vi "探头测量值显示.vi"(11 "校准参数":u16(ring) caption="校准参数：" items=["pH", "DO", "浊度", "电导率", "叶绿素a", "藻密度", "ORP", "COD", "DO2", "氯化物", "氨氮"]) -> (0 "线性系数":cluster{bool, "K":sgl, "B":sgl}, 1 "信号值":sgl, 2 "检测值":sgl, 3 "序列号":string, 4 "检测值.格式字符串":string, 5 "温度补偿系数":cluster{bool, "温度补偿系数":sgl}, 6 "信号值.格式字符串":string, 7 "电极状态标志":u16)   [LabVIEW 2016, in "斯坦道多参数.lvlib"]
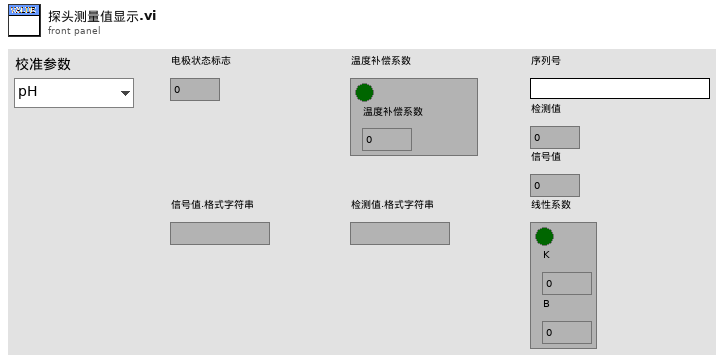
[diagram p1: front panel]
types:
  T1 = typedef "斯坦道多参数.lvlib/探头类型.ctl" = enum16{"禹山", "国弘", "纳清", "STD"}
  T2 = cluster{"pH探头选择":T1, "DO探头选择":T1, "电导率探头选择":T1, "浊度探头选择":T1, "叶绿素a探头选择":T1, "蓝绿藻探头选择":T1, "orp探头选择":T1, "COD探头选择":T1, "DO2探头选择":T1, "氨氮探头选择":T1, "水中油探头选择":T1}
  T3 = enum16{"null", "pH", "DO", "浊度", "电导率", "叶绿素a", "DO2"}
  T4 = enum16{"null", "pH", "DO", "浊度", "电导率", "叶绿素a", "DO2", "藻密度"}
  T5 = cluster{"输出值":cluster{"K":sgl, "B":sgl}, "SN":string}
  T6 = cluster{"电极状态标志":u16, "电极型号标志":u16, "酸碱度测量值":sgl, "温度测量值":sgl, "酸碱度信号值":sgl, "温度信号值":sgl, "酸碱度偏移修正值":sgl, "温度偏移修正值":sgl, "手动温度补偿值":sgl, "酸碱度电极零点":sgl, "酸碱度电极斜率":sgl, "第1点标准值记录":sgl, "第1点信号值记录":sgl, "第1点温度值记录":sgl, "第2点标准值记录":sgl, "第2点信号值记录":sgl, "第2点温度值记录":sgl, "命令滤波设定":u16, "温度模式":enum16{"ATC", "MTC"}, "生产批次":u16, "电极序号":u16, "串口地址":u16, "串口波特率":enum16{"9600", "19200", "115200"}, "串口校验位":enum16{"NONE", "ODD", "EVEN"}, "串口停止位":enum16{"1bit", "2bit"}, "第一点标准值":sgl, "第二点标准值":sgl}
  T7 = cluster{"报警码":u16, "pH数值":sgl, "0X0003_NC":sgl, "温度数据":sgl, "pH原始信号 mv":sgl, "0X0009_NC":string, "产品名称":string, "序列号":string, "硬件版本":string, "软件版本":string, "通讯地址":u16, "波特率":u16, "设备类型":u16, "0X0026_NC":string, "第一点原始数据":sgl, "第一点校准数据":sgl, "第二点原始数据":sgl, "第二点校准数据":sgl, "探头校准命令":u16, "温度校准参数":sgl, "温度校准命令":u16}
  T8 = cluster{"电极状态标志":u16, "电极型号标志":u16, "溶解氧测量值":sgl, "温度测量值":sgl, "溶解氧饱和度值":sgl, "盐度补偿值":sgl, "大气压补偿值":sgl, "溶解氧偏移修正值":sgl, "温度偏移修正值":sgl, "手动温度补偿值":sgl, "溶解氧电极零点":sgl, "溶解氧电极斜率":sgl, "第1点标准值记录":sgl, "第1点信号值记录":sgl, "第1点温度值记录":sgl, "第2点标准值记录":sgl, "第2点信号值记录":sgl, "第2点温度值记录":sgl, "命令滤波设定":u16, "温度模式":enum16{"ATC", "MTC"}, "生产批次":u16, "电极序号":u16, "串口地址":u16, "串口波特率":enum16{"9600", "19200", "115200"}, "串口校验位":enum16{"NONE", "ODD", "EVEN"}, "串口停止位":enum16{"1bit", "2bit"}, "第一点标准值":sgl, "第二点标准值":sgl}
  T9 = cluster{"报警码":u16, "溶解氧数值（mg/L）":sgl, "溶解氧数据（%）":sgl, "温度数据":sgl, "溶解氧原始信号 nA":sgl, "大气压力":sgl, "盐度":sgl, "0X0009_NC":string, "产品名称":string, "序列号":string, "硬件版本":string, "软件版本":string, "通讯地址":u16, "波特率":u16, "设备类型":u16, "0X0026_NC":string, "第一点原始数据":sgl, "第一点校准数据":sgl, "第二点原始数据":sgl, "第二点校准数据":sgl, "探头校准命令":u16, "温度校准参数":sgl, "温度校准命令":u16}
  T10 = cluster{"电极状态标志":u16, "电极型号标志":u16, "浊度测量值":sgl, "温度测量值":sgl, "浊度信号值":sgl, "浊度偏移修正值":sgl, "温度偏移修正值":sgl, "手动温度补偿值":sgl, "浊度电极零点":sgl, "浊度电极斜率":sgl, "清洁周期":u16, "命令滤波设定":u16, "温度模式":enum16{"ATC", "MTC"}, "生产批次":u16, "电极序号":u16, "串口地址":u16, "串口波特率":enum16{"9600", "19200", "115200"}, "串口校验位":enum16{"NONE", "ODD", "EVEN"}, "串口停止位":enum16{"1bit", "2bit"}, "第一点标准值":sgl, "第二点标准值":sgl, "第三点标准值":sgl}
  T11 = cluster{"报警码":u16, "浊度数值 NTU":sgl, "温度数据":sgl, "原始光强数值":u16, "量程":u16, "平均次数":u16, "清扫模式":u16, "清扫次数":u16, "清扫间隔分钟":u16, "0X000B_NC":string, "产品名称":string, "序列号":string, "硬件版本":string, "软件版本":string, "通讯地址":u16, "波特率":u16, "设备类型":u16, "0X0026_NC":string, "校准量程":u16, "第一点原始光强":u16, "第一点校准数据":sgl, "第二点原始光强":u16, "第二点校准数据":sgl, "第三点原始光强":u16, "第三点校准数据":sgl, "探头校准命令":u16, "温度校准参数":sgl, "温度校准命令":u16}
  T12 = cluster{"电极状态标志":u16, "电极型号标志":u16, "电导率测量值":sgl, "温度测量值":sgl, "电导率信号值":sgl, "温度信号值":sgl, "温度补偿系数":sgl, "电导率偏移修正值":sgl, "温度偏移修正值":sgl, "手动温度补偿值":sgl, "电导率电极零点":sgl, "电导率电极斜率":sgl, "命令滤波设定":u16, "温度模式":enum16{"ATC", "MTC"}, "生产批次":u16, "电极序号":u16, "串口地址":u16, "串口波特率":enum16{"9600", "19200", "115200"}, "串口校验位":enum16{"NONE", "ODD", "EVEN"}, "串口停止位":enum16{"1bit", "2bit"}, "第一点标准值":sgl, "第二点标准值":sgl}
  T13 = cluster{"报警码":u16, "电导率数据（uS/cm）":sgl, "0x0003 NC":sgl, "温度数据":sgl, "电导率原始信号电阻":sgl, "当前量程":u16, "温度补偿系数":sgl, "0X0009_NC":string, "产品名称":string, "序列号":string, "硬件版本":string, "软件版本":string, "通讯地址":u16, "波特率":u16, "设备类型":u16, "0X0026_NC":string, "第一点原始数据":sgl, "第一点校准数据":sgl, "0X0035_NC":sgl, "0X0037_NC":sgl, "探头校准命令":u16, "温度校准参数":sgl, "温度校准命令":u16}
  T14 = cluster{"报警码":u16, "叶绿素a":sgl, "温度数据":sgl, "原始光强数值":u16, "量程":u16, "平均次数":u16, "清扫模式":u16, "清扫次数":u16, "清扫间隔分钟":u16, "0X000B_NC":string, "产品名称":string, "序列号":string, "硬件版本":string, "软件版本":string, "通讯地址":u16, "波特率":u16, "设备类型":u16, "0X0026_NC":string, "校准量程":u16, "第一点原始光强":u16, "第一点校准数据":sgl, "第二点原始光强":u16, "第二点校准数据":sgl, "第三点原始光强":u16, "第三点校准数据":sgl, "探头校准命令":u16, "温度校准参数":sgl, "温度校准命令":u16}
  T15 = cluster{"报警码":u16, "蓝绿藻":sgl, "温度数据":sgl, "原始光强数值":u16, "量程":u16, "平均次数":u16, "清扫模式":u16, "清扫次数":u16, "清扫间隔分钟":u16, "0X000B_NC":string, "产品名称":string, "序列号":string, "硬件版本":string, "软件版本":string, "通讯地址":u16, "波特率":u16, "设备类型":u16, "0X0026_NC":string, "校准量程":u16, "第一点原始光强":u16, "第一点校准数据":sgl, "第二点原始光强":u16, "第二点校准数据":sgl, "第三点原始光强":u16, "第三点校准数据":sgl, "探头校准命令":u16, "温度校准参数":sgl, "温度校准命令":u16}
  T16 = cluster{"电极状态标志":u16, "电极型号标志":u16, "测量值":sgl, "温度测量值":sgl, "信号值":sgl, "温度信号值":sgl, "000AH_NC":sgl, "偏移修正值":sgl, "温度偏移修正值":sgl, "手动温度补偿值":sgl, "命令滤波设定":u16, "温度模式":enum16{"ATC", "MTC"}, "生产批次":u16, "传感器序号":u16, "串口地址":u16, "串口波特率":enum16{"9600", "19200", "115200"}, "串口校验位":enum16{"NONE", "ODD", "EVEN"}, "串口停止位":enum16{"1bit", "2bit"}}
  T17 = cluster{"电极状态标志":u16, "电极型号标志":u16, "COD测量值":sgl, "浊度测量值":sgl, "COD信号值":sgl, "浊度信号值":sgl, "温度测量值":sgl, "COD偏移修正值":sgl, "浊度偏移修正值":sgl, "COD水样校正值":sgl, "温度偏移修正值":sgl, "COD零点系数":sgl, "COD斜率系数":sgl, "浊度零点系数":sgl, "浊度斜率系数":sgl, "COD测值K值":sgl, "浊度测值K值":sgl, "浊度补偿COD系数值":sgl, "COD温度补偿系数值 ":sgl, "测量周期":u16, "清洗周期":u16, "命令寄存器":u16, "数字滤波设定":u16, "温度模式":enum16{"AUTO", "OFF"}, "生产批次":u16, "电极序号":u16, "串口地址":u16, "串口波特率":enum16{"9600", "19200", "115200"}, "串口校验位":enum16{"NONE", "ODD", "EVEN"}, "串口停止位":enum16{"1bit", "2bit"}, "第一点校正指令":u16, "第一点标准值":sgl, "第二点校正指令":u16, "第二点标准值":sgl, "第三点校正指令":u16, "第三点标准值":sgl, "COD吸光度":sgl, "浊度吸光度":sgl, "温度信号值":sgl}
  T18 = cluster{"电极状态标志":u16, "电极型号标志":u16, "测量值":sgl, "温度测量值":sgl, "信号值":sgl, "温度信号值":sgl, "偏移修正值":sgl, "温度偏移修正值":sgl, "手动温度补偿值":sgl, "电极零点":sgl, "电极斜率":sgl, "第1点标准值记录":sgl, "第1点信号值记录":sgl, "第1点温度值记录":sgl, "第2点标准值记录":sgl, "第2点信号值记录":sgl, "第2点温度值记录":sgl, "命令滤波设定":u16, "温度模式":enum16{"ATC", "MTC"}, "生产批次":u16, "电极序号":u16, "串口地址":u16, "串口波特率":enum16{"9600", "19200", "115200"}, "串口校验位":enum16{"NONE", "ODD", "EVEN"}, "串口停止位":enum16{"1bit", "2bit"}, "第一点标准值":sgl, "第二点标准值":sgl}
  T19 = cluster{"报警码":u16, "参数1数据":sgl, "参数2数据":sgl, "参数3数据":sgl, "参数4数据":sgl, "温度数据":sgl, "参数1原始信号":sgl, "参数2原始信号":sgl, "参数3原始信号":sgl, "参数4原始信号":sgl, "序列号":string, "硬件版本":string, "软件版本":string, "通讯地址":u16, "波特率":u16, "设备类型":u16, "0X0026_NC":string, "校准参数类型":u16, "第一点原始数据":sgl, "第一点校准数据":sgl, "第二点原始数据":sgl, "第二点校准数据":sgl, "探头校准命令":u16, "温度校准参数":sgl, "温度校准命令":u16}
  T20 = cluster{"电极状态标志":u16, "电极型号标志":u16, "测量值":sgl, "温度测量值":sgl, "信号值":sgl, "水中油B值":sgl, "温度B值":sgl, "水中油零点系数":sgl, "水中油斜率系数":sgl, "水中油K值":sgl, "空白电位值":sgl, "温度信号值":sgl, "温度补偿系数":sgl, "测量档位":u16, "清洁周期":u16, "命令寄存器":u16, "数位滤波设定":u16, "温度模式":enum16{"ATC", "MTC"}, "生产批次":u16, "电极序号":u16, "串口地址":u16, "串口波特率":enum16{"9600", "19200", "115200"}, "串口校验位":enum16{"NONE", "ODD", "EVEN"}, "串口停止位":enum16{"1bit", "2bit"}, "第一点校正指令":u16, "第一点标准值":sgl, "第二点校正指令":u16, "第二点标准值":sgl, "第三点校正指令":u16, "第三点标准值":sgl}
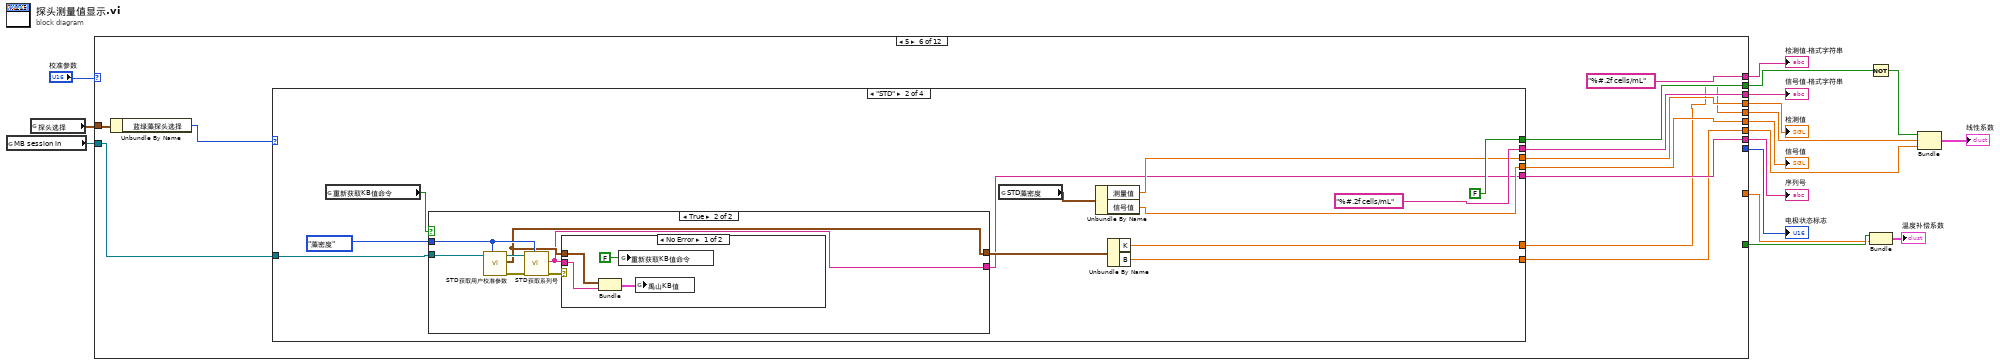
[diagram p0: block diagram]
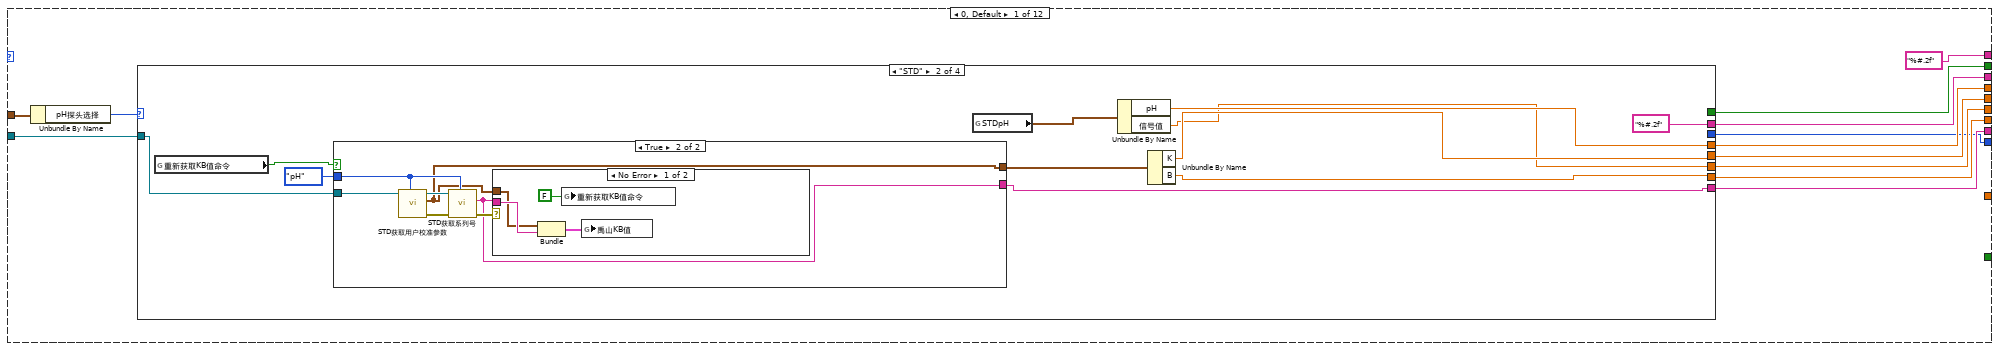
[diagram p2: hidden frame]
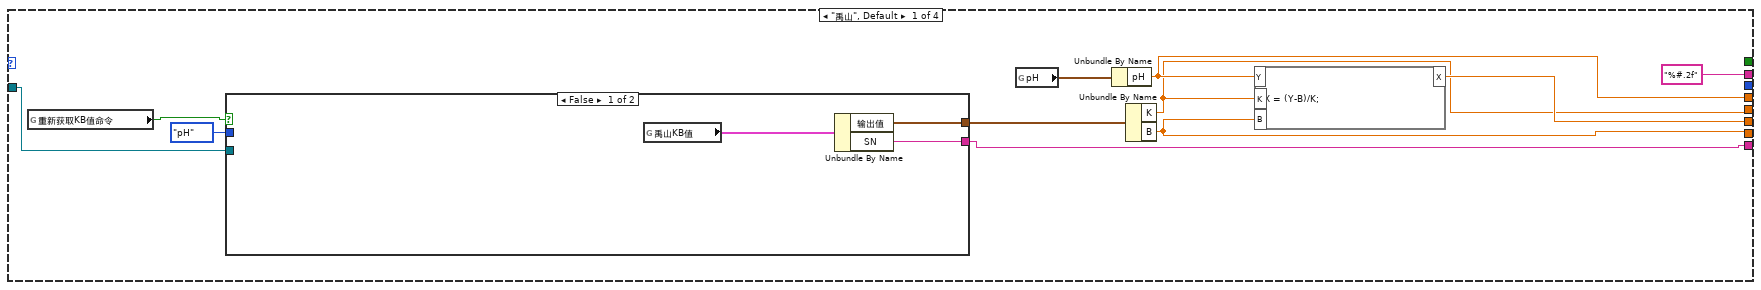
[diagram p3: hidden frame]
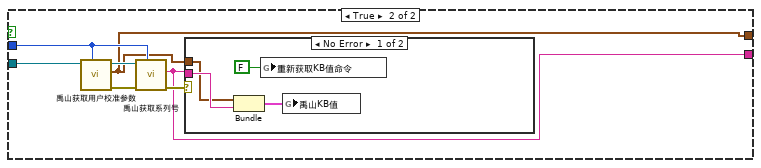
[diagram p4: hidden frame]
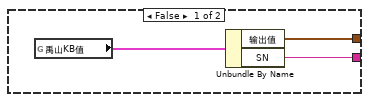
[diagram p6: hidden frame]
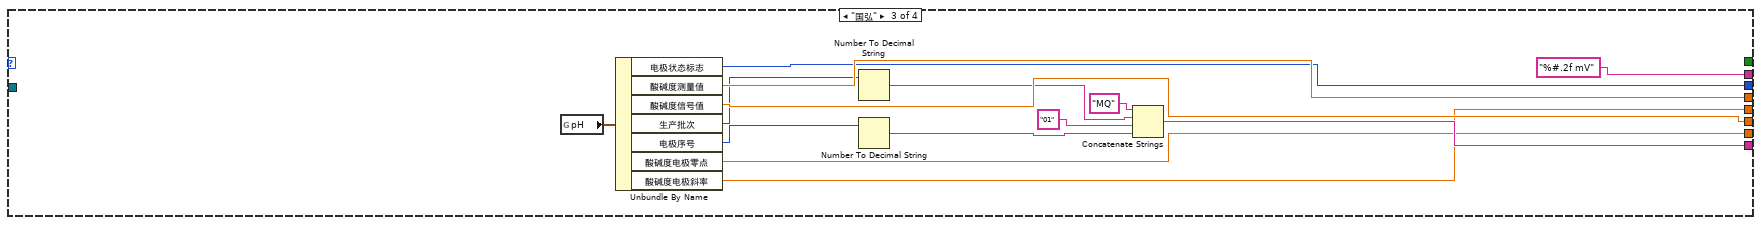
[diagram p8: hidden frame]
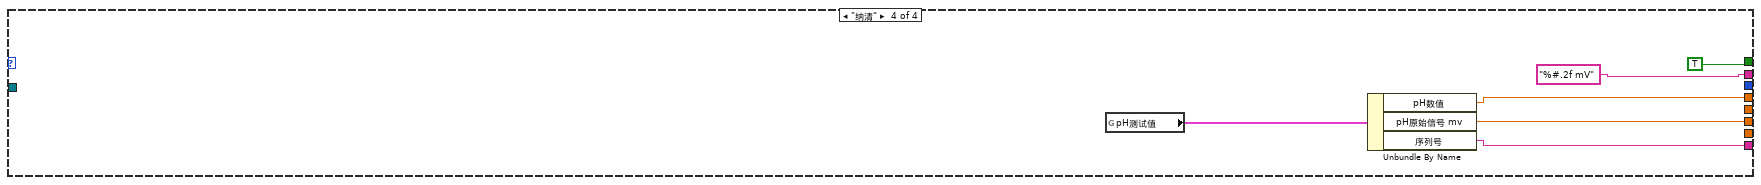
[diagram p9: hidden frame]
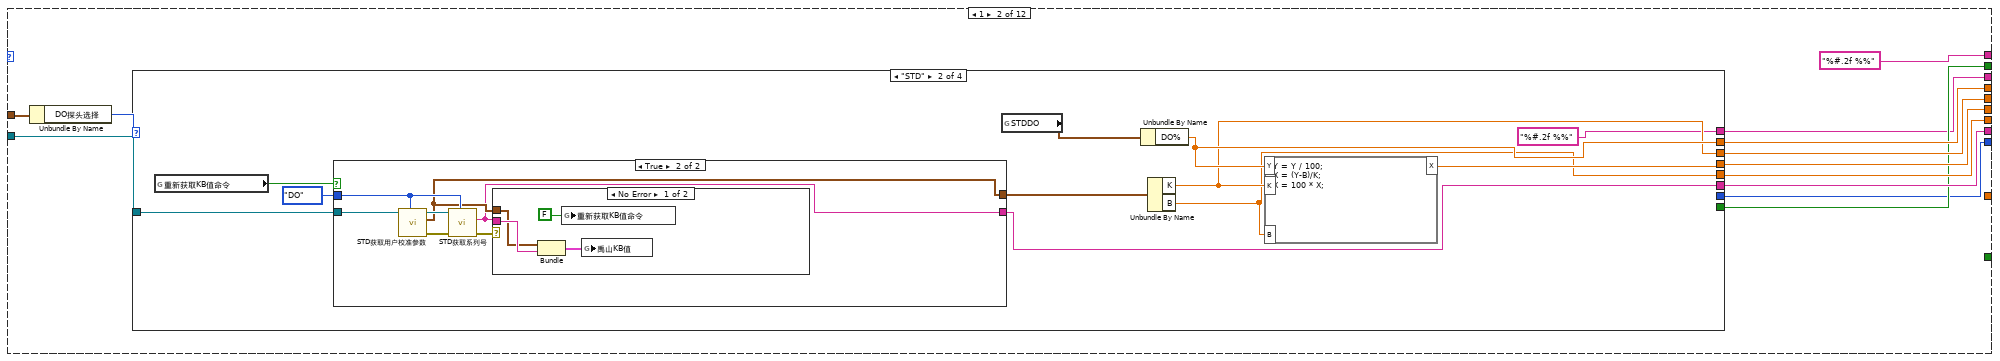
[diagram p10: hidden frame]
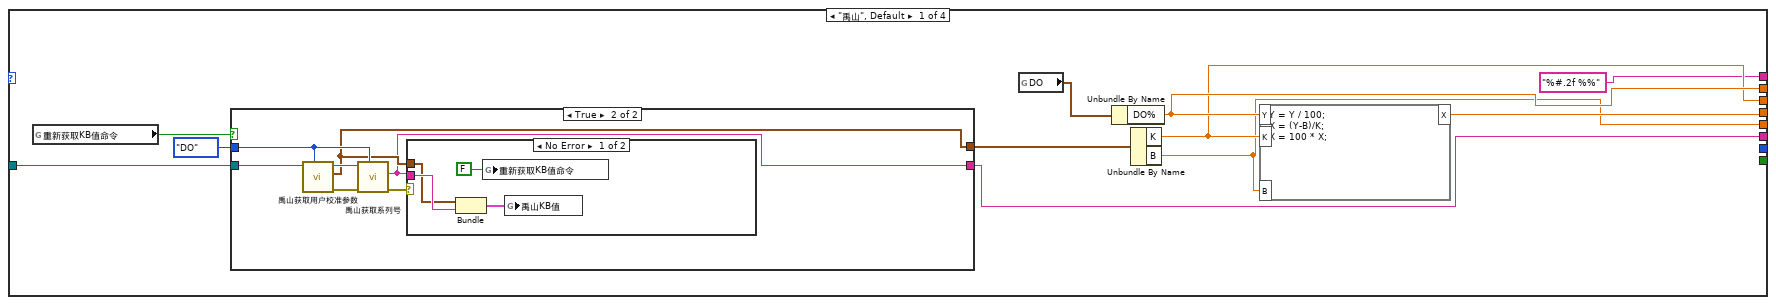
[diagram p11: hidden frame]
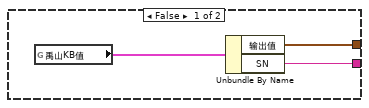
[diagram p12: hidden frame]
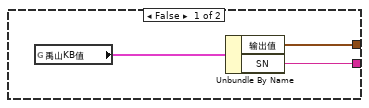
[diagram p14: hidden frame]
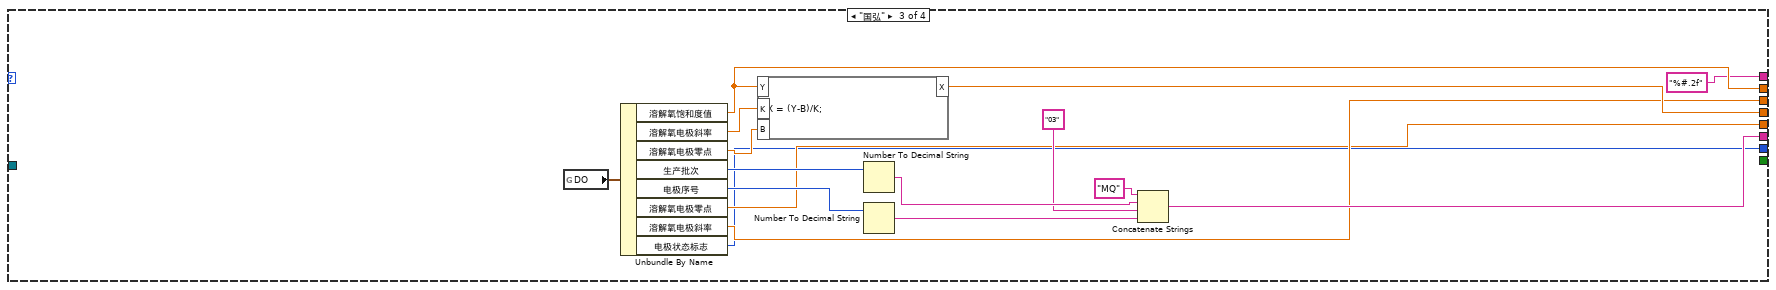
[diagram p16: hidden frame]
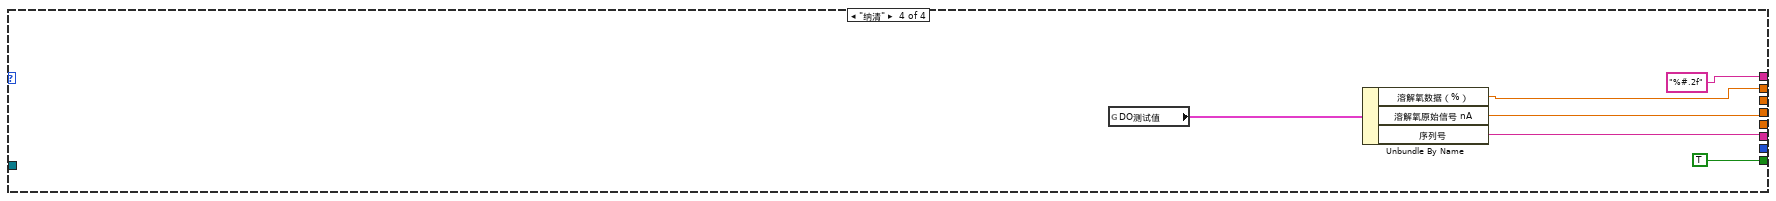
[diagram p17: hidden frame]
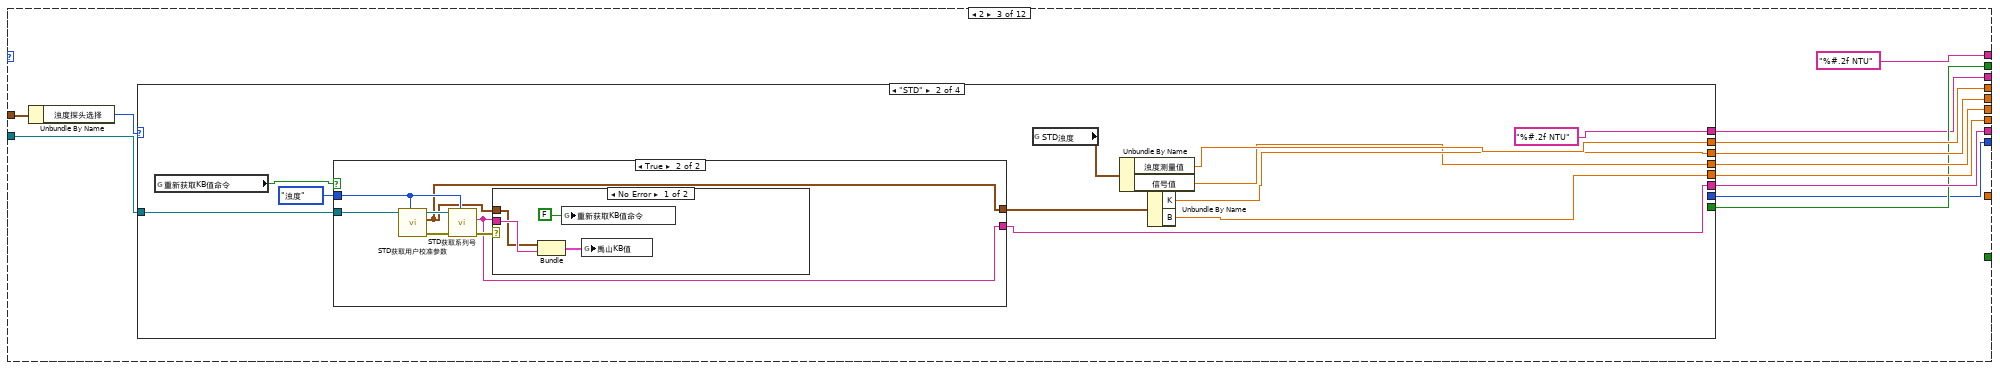
[diagram p18: hidden frame]
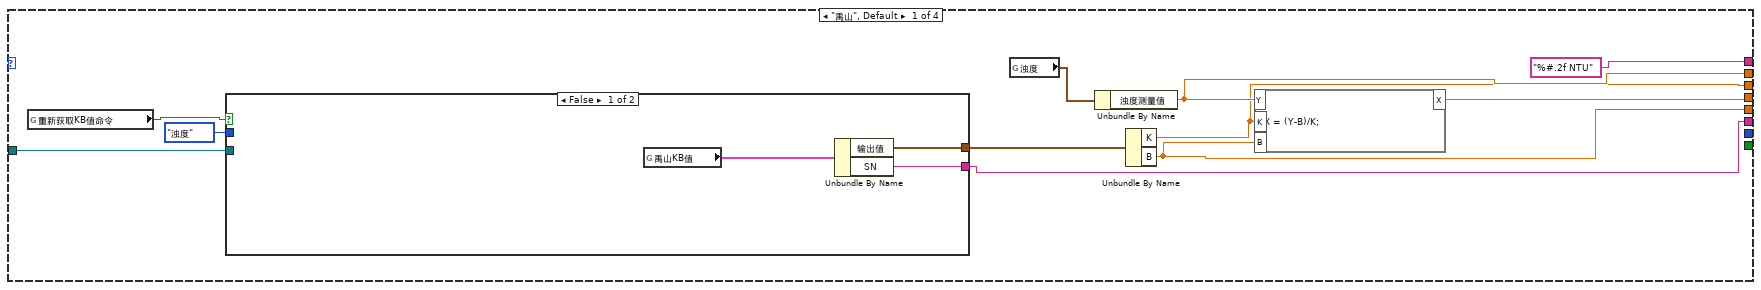
[diagram p19: hidden frame]
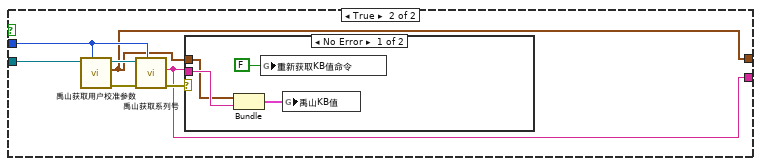
[diagram p20: hidden frame]
diagram:
  n1 = global read "多参数全局变量.vi" "MB session in"() -> (w13:refnum<class "MB_Master.lvclass">)
  n2 = global read "断电保存变量.vi" "探头选择"() -> (w15:T2)
  n3 = case shown="5" "校准参数" {
    tunnel: [w28 w110 w194 w278 w363 w434 w485 w519 w530 w561 w568 w583] -> w17
    tunnel: w15 -> [w27 w109 w193 w277 w362 w433 w484 _ _ _ _ _]
    tunnel: [w26 w108 w192 w276 w361 w432 w483 w518 w531 w560 w567 w582] -> w14
    tunnel: w13 -> [w25 w107 w191 w275 w360 w427 _ _ w528 _ _ _]
    tunnel: [w24 w106 w190 w274 w359 w431 w482 w517 w529 w559 w566 w581] -> w12
    tunnel: [w23 w105 w189 w273 w358 w426 sgl 0.0 ("K") w516 w524 w558 _ w580] -> w9
    tunnel: [w22 w104 w188 w272 w357 w425 sgl 0.0 ("B") w515 w523 w557 _ w579] -> w8
    tunnel: [w21 w103 w187 w271 w356 w430 w481 _ FALSE _ TRUE _] -> w11
    tunnel: ["%#.2f" ("数值文本.格式字符串") "%#.2f %%" ("数值文本.格式字符串") "%#.2f NTU" ("数值文本.格式字符串") "%#.2f μS/cm" ("数值文本.格式字符串") "%#.2f μg/L" ("数值文本.格式字符串") "%#.2f cells/mL" ("数值文本.格式字符串") "%#.2f mV" ("数值文本.格式字符串") "%#.2f" ("数值文本.格式字符串") "%#.2f %%" ("数值文本.格式字符串") "%#.2f" ("数值文本.格式字符串") "%#.2f" ("数值文本.格式字符串") "%#.2f" ("数值文本.格式字符串")] -> w6
    tunnel: [_ _ _ w269 _ _ _ _ _ _ _ _] -> w4
    tunnel: [_ _ _ w268 _ _ _ _ _ _ _ _] -> w5
    tunnel: [w19 w101 w185 w267 _ _ w477 w513 _ w555 _ w577] -> w2
    tunnel: [w18 w100 w184 w266 w354 w428 "%#.2f mV" ("数值文本.格式字符串") "%#.2f mV" ("数值文本.格式字符串") "%#.2f %%" ("数值文本.格式字符串") "%#.2f mV" ("数值文本.格式字符串") "%#.2f mV" ("数值文本.格式字符串") "%#.2f mV" ("数值文本.格式字符串")] -> w1
    frame 0, Default {
      n4 = Unbundle By Name(w27) -> ("pH探头选择"=w29:T1)
      n5 = case shown="\"STD\"" w29 {
        tunnel: [w39 w64 w92 w99] -> w28
        tunnel: [w38 w55 w91 w97] -> w26
        tunnel: w25 -> [w36 w62 _ _]
        tunnel: [w37 w63 w84 w96] -> w24
        tunnel: [w33 w59 w83 _] -> w23
        tunnel: [w32 w58 w82 _] -> w22
        tunnel: [_ _ _ TRUE] -> w21
        tunnel: [_ _ w81 _] -> w19
        tunnel: ["%#.2f" ("数值文本.格式字符串") "%#.2f" ("数值文本.格式字符串") "%#.2f mV" ("数值文本.格式字符串") "%#.2f mV" ("数值文本.格式字符串")] -> w18
        frame "禹山", Default {
          n6 = global read "多参数全局变量.vi" "重新获取KB值命令"() -> (w30:bool)
          n7 = case shown="False" w30 {
            tunnel: [w41 w45] -> w37
            tunnel: w36 -> [_ w50]
            tunnel: T3."pH" ("探头") -> [_ w49]
            tunnel: [w42 w44] -> w34
            frame False {
              n8 = global read "多参数全局变量.vi" "禹山KB值"() -> (w43:T5)
              n9 = Unbundle By Name(w43) -> ("输出值"=w42:cluster{"K":sgl, "B":sgl}, "SN"=w41:string)
            }
            frame True {
              n10 = call "禹山获取用户校准参数.vi"("探头"=w49, "MB session in"=w50) -> ("error out"=w47:errorcluster, "输出值"=w44:cluster{"K":sgl, "B":sgl}, "MB session out"=w48:refnum<class "MB_Master.lvclass">)  [unwired: 7 in]
              n11 = call "禹山获取系列号.vi"("探头"=w49, "error in (no error)"=w47, "MB session in"=w48) -> ("error out"=w46:errorcluster, "SN"=w45:string)  [unwired: 6 in, 1 out]
              n12 = case shown="No Error" w46 {
                tunnel: w44 -> [w53 _]
                tunnel: w45 -> [w54 _]
                frame No Error {
                  n13 = Bundle("输出值"=w53, "SN"=w54) -> (w52:T5)  [unwired: 1 in]
                  n14 = global write "多参数全局变量.vi" "重新获取KB值命令"(FALSE ("重新获取KB值命令")) -> ()
                  n15 = global write "多参数全局变量.vi" "禹山KB值"(w52) -> ()
                }
                frame Error {
                }
              }
            }
          }
          n16 = global read "禹山过程全局变量.vi" "pH"() -> (w40:cluster{"温度测量值":sgl, "ORP":sgl, "pH":sgl})
          n17 = Unbundle By Name(w40) -> ("pH"=w39:sgl)
          n18 = Unbundle By Name(w34) -> ("K"=w33:sgl, "B"=w32:sgl)
          n19 = formula code="X = (Y-B)/K;"("Y"=w39, "K"=w33, "B"=w32) -> ("X"=w38:dbl)
        }
        frame "STD" {
          n20 = global read "多参数全局变量.vi" "重新获取KB值命令"() -> (w56:bool)
          n21 = case shown="True" w56 {
            tunnel: [w66 w70] -> w63
            tunnel: w62 -> [_ w75]
            tunnel: T3."pH" ("探头") -> [_ w74]
            tunnel: [w67 w69] -> w60
            frame False {
              n22 = global read "多参数全局变量.vi" "禹山KB值"() -> (w68:T5)
              n23 = Unbundle By Name(w68) -> ("输出值"=w67:cluster{"K":sgl, "B":sgl}, "SN"=w66:string)
            }
            frame True {
              n24 = call "STD获取用户校准参数.vi"("探头"=w74, "MB session in"=w75) -> ("error out"=w72:errorcluster, "输出值"=w69:cluster{"K":sgl, "B":sgl}, "MB session out"=w73:refnum<class "MB_Master.lvclass">)  [unwired: 7 in]
              n25 = call "STD获取系列号.vi"("探头"=w74, "error in (no error)"=w72, "MB session in"=w73) -> ("error out"=w71:errorcluster, "SN"=w70:string)  [unwired: 6 in, 1 out]
              n26 = case shown="No Error" w71 {
                tunnel: w69 -> [w78 _]
                tunnel: w70 -> [w79 _]
                frame No Error {
                  n27 = Bundle("输出值"=w78, "SN"=w79) -> (w77:T5)  [unwired: 1 in]
                  n28 = global write "多参数全局变量.vi" "重新获取KB值命令"(FALSE ("重新获取KB值命令")) -> ()
                  n29 = global write "多参数全局变量.vi" "禹山KB值"(w77) -> ()
                }
                frame Error {
                }
              }
            }
          }
          n30 = global read "禹山过程全局变量.vi" "STDpH"() -> (w65:cluster{"温度测量值":sgl, "pH":sgl, "信号值":sgl})
          n31 = Unbundle By Name(w65) -> ("pH"=w64:sgl, "信号值"=w55:sgl)
          n32 = Unbundle By Name(w60) -> ("K"=w59:sgl, "B"=w58:sgl)
        }
        frame "国弘" {
          n33 = global read "国弘过程全局变量.vi" "pH"() -> (w93:T6)
          n34 = Unbundle By Name(w93) -> ("电极状态标志"=w81:u16, "酸碱度测量值"=w92:sgl, "酸碱度信号值"=w91:sgl, "生产批次"=w86:u16, "电极序号"=w85:u16, "酸碱度电极零点"=w82:sgl, "酸碱度电极斜率"=w83:sgl)
          n35 = Number To Decimal String(number=w86) -> (decimal integer string=w90:string)  [unwired: 1 in]
          n36 = Number To Decimal String(number=w85) -> (decimal integer string=w88:string)  [unwired: 1 in]
          n37 = Concatenate Strings("MQ" ("字符串"), w90, "01" ("字符串"), w88) -> (w84:string)
        }
        frame "纳清" {
          n38 = global read "纳清过程全局变量.vi" "pH测试值"() -> (w98:T7)
          n39 = Unbundle By Name(w98) -> ("pH数值"=w99:sgl, "pH原始信号 mv"=w97:sgl, "序列号"=w96:string)
        }
      }
    }
    frame 1 {
      n40 = Unbundle By Name(w109) -> ("DO探头选择"=w111:T1)
      n41 = case shown="\"STD\"" w111 {
        tunnel: [w121 w146 w175 w183] -> w110
        tunnel: [w120 w145 w173 w181] -> w108
        tunnel: w107 -> [w118 w143 _ _]
        tunnel: [w119 w144 w166 w180] -> w106
        tunnel: [w115 w140 w165 _] -> w105
        tunnel: [w114 w139 w164 _] -> w104
        tunnel: [_ _ _ TRUE] -> w103
        tunnel: [_ _ w163 _] -> w101
        tunnel: ["%#.2f %%" ("数值文本.格式字符串") "%#.2f %%" ("数值文本.格式字符串") "%#.2f" ("数值文本.格式字符串") "%#.2f" ("数值文本.格式字符串")] -> w100
        frame "禹山", Default {
          n42 = global read "多参数全局变量.vi" "重新获取KB值命令"() -> (w112:bool)
          n43 = case shown="True" w112 {
            tunnel: [w123 w126] -> w119
            tunnel: w118 -> [_ w132]
            tunnel: [w124 w127] -> w117
            tunnel: T3."DO" ("探头") -> [_ w129]
            frame False {
              n44 = global read "多参数全局变量.vi" "禹山KB值"() -> (w125:T5)
              n45 = Unbundle By Name(w125) -> ("输出值"=w124:cluster{"K":sgl, "B":sgl}, "SN"=w123:string)
            }
            frame True {
              n46 = call "禹山获取用户校准参数.vi"("探头"=w129, "MB session in"=w132) -> ("error out"=w131:errorcluster, "输出值"=w127:cluster{"K":sgl, "B":sgl}, "MB session out"=w130:refnum<class "MB_Master.lvclass">)  [unwired: 7 in]
              n47 = call "禹山获取系列号.vi"("探头"=w129, "error in (no error)"=w131, "MB session in"=w130) -> ("error out"=w128:errorcluster, "SN"=w126:string)  [unwired: 6 in, 1 out]
              n48 = case shown="No Error" w128 {
                tunnel: w127 -> [w135 _]
                tunnel: w126 -> [w136 _]
                frame No Error {
                  n49 = Bundle("输出值"=w135, "SN"=w136) -> (w134:T5)  [unwired: 1 in]
                  n50 = global write "多参数全局变量.vi" "重新获取KB值命令"(FALSE ("重新获取KB值命令")) -> ()
                  n51 = global write "多参数全局变量.vi" "禹山KB值"(w134) -> ()
                }
                frame Error {
                }
              }
            }
          }
          n52 = global read "禹山过程全局变量.vi" "DO"() -> (w122:cluster{"温度测量值":sgl, "DO%":sgl, "DOmg/L":sgl})
          n53 = Unbundle By Name(w122) -> ("DO%"=w121:sgl)
          n54 = Unbundle By Name(w117) -> ("K"=w115:sgl, "B"=w114:sgl)
          n55 = formula code="Y = Y / 100;\nX = (Y-B)/K;\nX = 100 * X;"("Y"=w121, "K"=w115, "B"=w114) -> ("X"=w120:dbl)
        }
        frame "STD" {
          n56 = global read "多参数全局变量.vi" "重新获取KB值命令"() -> (w137:bool)
          n57 = case shown="True" w137 {
            tunnel: [w148 w151] -> w144
            tunnel: w143 -> [_ w157]
            tunnel: [w149 w152] -> w142
            tunnel: T3."DO" ("探头") -> [_ w154]
            frame False {
              n58 = global read "多参数全局变量.vi" "禹山KB值"() -> (w150:T5)
              n59 = Unbundle By Name(w150) -> ("输出值"=w149:cluster{"K":sgl, "B":sgl}, "SN"=w148:string)
            }
            frame True {
              n60 = call "STD获取用户校准参数.vi"("探头"=w154, "MB session in"=w157) -> ("error out"=w156:errorcluster, "输出值"=w152:cluster{"K":sgl, "B":sgl}, "MB session out"=w155:refnum<class "MB_Master.lvclass">)  [unwired: 7 in]
              n61 = call "STD获取系列号.vi"("探头"=w154, "error in (no error)"=w156, "MB session in"=w155) -> ("error out"=w153:errorcluster, "SN"=w151:string)  [unwired: 6 in, 1 out]
              n62 = case shown="No Error" w153 {
                tunnel: w152 -> [w160 _]
                tunnel: w151 -> [w161 _]
                frame No Error {
                  n63 = Bundle("输出值"=w160, "SN"=w161) -> (w159:T5)  [unwired: 1 in]
                  n64 = global write "多参数全局变量.vi" "重新获取KB值命令"(FALSE ("重新获取KB值命令")) -> ()
                  n65 = global write "多参数全局变量.vi" "禹山KB值"(w159) -> ()
                }
                frame Error {
                }
              }
            }
          }
          n66 = global read "禹山过程全局变量.vi" "STDDO"() -> (w147:cluster{"温度测量值":sgl, "DO%":sgl, "DOmg/L":sgl})
          n67 = Unbundle By Name(w147) -> ("DO%"=w146:sgl)
          n68 = Unbundle By Name(w142) -> ("K"=w140:sgl, "B"=w139:sgl)
          n69 = formula code="Y = Y / 100;\nX = (Y-B)/K;\nX = 100 * X;"("Y"=w146, "K"=w140, "B"=w139) -> ("X"=w145:dbl)
        }
        frame "国弘" {
          n70 = global read "国弘过程全局变量.vi" "DO"() -> (w177:T8)
          n71 = Unbundle By Name(w177) -> ("溶解氧饱和度值"=w175:sgl, "溶解氧电极斜率"=w176:sgl, "溶解氧电极零点"=w174:sgl, "生产批次"=w167:u16, "电极序号"=w168:u16, "溶解氧电极零点"=w164:sgl, "溶解氧电极斜率"=w165:sgl, "电极状态标志"=w163:u16)
          n72 = formula code="X = (Y-B)/K;"("Y"=w175, "K"=w176, "B"=w174) -> ("X"=w173:dbl)
          n73 = Number To Decimal String(number=w167) -> (decimal integer string=w172:string)  [unwired: 1 in]
          n74 = Number To Decimal String(number=w168) -> (decimal integer string=w170:string)  [unwired: 1 in]
          n75 = Concatenate Strings("MQ" ("字符串"), w172, "03" ("字符串"), w170) -> (w166:string)
        }
        frame "纳清" {
          n76 = global read "纳清过程全局变量.vi" "DO测试值"() -> (w182:T9)
          n77 = Unbundle By Name(w182) -> ("溶解氧数据（%）"=w183:sgl, "溶解氧原始信号 nA"=w181:sgl, "序列号"=w180:string)
        }
      }
    }
    frame 2 {
      n78 = Unbundle By Name(w193) -> ("浊度探头选择"=w195:T1)
      n79 = case shown="\"STD\"" w195 {
        tunnel: [w205 w230 w258 w265] -> w194
        tunnel: [w204 w221 w257 w263] -> w192
        tunnel: w191 -> [w202 w228 _ _]
        tunnel: [w203 w229 w252 w262] -> w190
        tunnel: [w199 w225 w249 _] -> w189
        tunnel: [w198 w224 w248 _] -> w188
        tunnel: [_ _ _ TRUE] -> w187
        tunnel: [_ _ w247 _] -> w185
        tunnel: ["%#.2f NTU" ("数值文本.格式字符串") "%#.2f NTU" ("数值文本.格式字符串") "%#.2f NTU" ("数值文本.格式字符串") "%#.6f" ("数值文本.格式字符串")] -> w184
        frame "禹山", Default {
          n80 = global read "多参数全局变量.vi" "重新获取KB值命令"() -> (w196:bool)
          n81 = case shown="False" w196 {
            tunnel: [w207 w211] -> w203
            tunnel: w202 -> [_ w216]
            tunnel: [w208 w210] -> w201
            tunnel: T3."浊度" ("探头") -> [_ w213]
            frame False {
              n82 = global read "多参数全局变量.vi" "禹山KB值"() -> (w209:T5)
              n83 = Unbundle By Name(w209) -> ("输出值"=w208:cluster{"K":sgl, "B":sgl}, "SN"=w207:string)
            }
            frame True {
              n84 = call "禹山获取用户校准参数.vi"("探头"=w213, "MB session in"=w216) -> ("error out"=w214:errorcluster, "输出值"=w210:cluster{"K":sgl, "B":sgl}, "MB session out"=w215:refnum<class "MB_Master.lvclass">)  [unwired: 7 in]
              n85 = call "禹山获取系列号.vi"("探头"=w213, "error in (no error)"=w214, "MB session in"=w215) -> ("error out"=w212:errorcluster, "SN"=w211:string)  [unwired: 6 in, 1 out]
              n86 = case shown="No Error" w212 {
                tunnel: w210 -> [w219 _]
                tunnel: w211 -> [w220 _]
                frame No Error {
                  n87 = Bundle("输出值"=w219, "SN"=w220) -> (w218:T5)  [unwired: 1 in]
                  n88 = global write "多参数全局变量.vi" "重新获取KB值命令"(FALSE ("重新获取KB值命令")) -> ()
                  n89 = global write "多参数全局变量.vi" "禹山KB值"(w218) -> ()
                }
                frame Error {
                }
              }
            }
          }
          n90 = global read "禹山过程全局变量.vi" "浊度"() -> (w206:cluster{"温度测量值":sgl, "浊度测量值":sgl})
          n91 = Unbundle By Name(w206) -> ("浊度测量值"=w205:sgl)
          n92 = Unbundle By Name(w201) -> ("K"=w199:sgl, "B"=w198:sgl)
          n93 = formula code="X = (Y-B)/K;"("Y"=w205, "K"=w199, "B"=w198) -> ("X"=w204:dbl)
        }
        frame "STD" {
          n94 = global read "多参数全局变量.vi" "重新获取KB值命令"() -> (w222:bool)
          n95 = case shown="True" w222 {
            tunnel: [w232 w236] -> w229
            tunnel: w228 -> [_ w241]
            tunnel: [w233 w235] -> w227
            tunnel: T3."浊度" ("探头") -> [_ w238]
            frame False {
              n96 = global read "多参数全局变量.vi" "禹山KB值"() -> (w234:T5)
              n97 = Unbundle By Name(w234) -> ("输出值"=w233:cluster{"K":sgl, "B":sgl}, "SN"=w232:string)
            }
            frame True {
              n98 = call "STD获取用户校准参数.vi"("探头"=w238, "MB session in"=w241) -> ("error out"=w239:errorcluster, "输出值"=w235:cluster{"K":sgl, "B":sgl}, "MB session out"=w240:refnum<class "MB_Master.lvclass">)  [unwired: 7 in]
              n99 = call "STD获取系列号.vi"("探头"=w238, "error in (no error)"=w239, "MB session in"=w240) -> ("error out"=w237:errorcluster, "SN"=w236:string)  [unwired: 6 in, 1 out]
              n100 = case shown="No Error" w237 {
                tunnel: w235 -> [w244 _]
                tunnel: w236 -> [w245 _]
                frame No Error {
                  n101 = Bundle("输出值"=w244, "SN"=w245) -> (w243:T5)  [unwired: 1 in]
                  n102 = global write "多参数全局变量.vi" "重新获取KB值命令"(FALSE ("重新获取KB值命令")) -> ()
                  n103 = global write "多参数全局变量.vi" "禹山KB值"(w243) -> ()
                }
                frame Error {
                }
              }
            }
          }
          n104 = global read "禹山过程全局变量.vi" "STD浊度"() -> (w231:cluster{"温度测量值":sgl, "浊度测量值":sgl, "信号值":sgl})
          n105 = Unbundle By Name(w231) -> ("浊度测量值"=w230:sgl, "信号值"=w221:sgl)
          n106 = Unbundle By Name(w227) -> ("K"=w225:sgl, "B"=w224:sgl)
        }
        frame "国弘" {
          n107 = global read "国弘过程全局变量.vi" "Turb"() -> (w259:T10)
          n108 = Unbundle By Name(w259) -> ("浊度测量值"=w258:sgl, "浊度信号值"=w257:sgl, "生产批次"=w250:u16, "电极序号"=w251:u16, "浊度电极零点"=w248:sgl, "浊度电极斜率"=w249:sgl, "电极状态标志"=w247:u16)
          n109 = Number To Decimal String(number=w250) -> (decimal integer string=w256:string)  [unwired: 1 in]
          n110 = Number To Decimal String(number=w251) -> (decimal integer string=w254:string)  [unwired: 1 in]
          n111 = Concatenate Strings("MQ" ("字符串"), w256, "04" ("字符串"), w254) -> (w252:string)
        }
        frame "纳清" {
          n112 = global read "纳清过程全局变量.vi" "浊度测试值"() -> (w264:T11)
          n113 = Unbundle By Name(w264) -> ("浊度数值 NTU"=w265:sgl, "原始光强数值"=w263:u16, "序列号"=w262:string)
        }
      }
    }
    frame 3 {
      n114 = Unbundle By Name(w277) -> ("电导率探头选择"=w279:T1)
      n115 = case shown="\"STD\"" w279 {
        tunnel: [w283 w309 w344 w353] -> w278
        tunnel: [w289 w305 w343 w351] -> w276
        tunnel: w275 -> [w287 w313 _ _]
        tunnel: [w288 w314 w338 w350] -> w274
        tunnel: [w284 w310 w335 _] -> w273
        tunnel: [w281 w307 w334 _] -> w272
        tunnel: [_ _ _ TRUE] -> w271
        tunnel: [_ _ w333 w348] -> w269
        tunnel: [_ _ TRUE TRUE] -> w268
        tunnel: [_ _ w331 _] -> w267
        tunnel: ["%#.2f μS/cm" ("数值文本.格式字符串") "%#.2f μS/cm" ("数值文本.格式字符串") "%#.2f μS/cm" ("数值文本.格式字符串") "%#.6f" ("数值文本.格式字符串")] -> w266
        frame "禹山", Default {
          n116 = global read "多参数全局变量.vi" "重新获取KB值命令"() -> (w280:bool)
          n117 = case shown="False" w280 {
            tunnel: [w291 w295] -> w288
            tunnel: w287 -> [_ w300]
            tunnel: [w292 w294] -> w286
            tunnel: T3."电导率" ("探头") -> [_ w297]
            frame False {
              n118 = global read "多参数全局变量.vi" "禹山KB值"() -> (w293:T5)
              n119 = Unbundle By Name(w293) -> ("输出值"=w292:cluster{"K":sgl, "B":sgl}, "SN"=w291:string)
            }
            frame True {
              n120 = call "禹山获取用户校准参数.vi"("探头"=w297, "MB session in"=w300) -> ("error out"=w299:errorcluster, "输出值"=w294:cluster{"K":sgl, "B":sgl}, "MB session out"=w298:refnum<class "MB_Master.lvclass">)  [unwired: 7 in]
              n121 = call "禹山获取系列号.vi"("探头"=w297, "error in (no error)"=w299, "MB session in"=w298) -> ("error out"=w296:errorcluster, "SN"=w295:string)  [unwired: 6 in, 1 out]
              n122 = case shown="No Error" w296 {
                tunnel: w294 -> [w303 _]
                tunnel: w295 -> [w304 _]
                frame No Error {
                  n123 = Bundle("输出值"=w303, "SN"=w304) -> (w302:T5)  [unwired: 1 in]
                  n124 = global write "多参数全局变量.vi" "重新获取KB值命令"(FALSE ("重新获取KB值命令")) -> ()
                  n125 = global write "多参数全局变量.vi" "禹山KB值"(w302) -> ()
                }
                frame Error {
                }
              }
            }
          }
          n126 = global read "禹山过程全局变量.vi" "spcond"() -> (w290:cluster{"温度测量值":sgl, "测量值":sgl, "错误标志":u16})
          n127 = Unbundle By Name(w290) -> ("测量值"=w283:sgl)
          n128 = Unbundle By Name(w286) -> ("K"=w284:sgl, "B"=w281:sgl)
          n129 = formula code="Y=Y/1000;\nX = (Y-B)/K;\nX=X*1000;"("Y"=w283, "K"=w284, "B"=w281) -> ("X"=w289:dbl)
        }
        frame "STD" {
          n130 = global read "多参数全局变量.vi" "重新获取KB值命令"() -> (w306:bool)
          n131 = case shown="True" w306 {
            tunnel: [w316 w320] -> w314
            tunnel: w313 -> [_ w325]
            tunnel: [w317 w319] -> w312
            tunnel: T3."电导率" ("探头") -> [_ w322]
            frame False {
              n132 = global read "多参数全局变量.vi" "禹山KB值"() -> (w318:T5)
              n133 = Unbundle By Name(w318) -> ("输出值"=w317:cluster{"K":sgl, "B":sgl}, "SN"=w316:string)
            }
            frame True {
              n134 = call "STD获取用户校准参数.vi"("探头"=w322, "MB session in"=w325) -> ("error out"=w324:errorcluster, "输出值"=w319:cluster{"K":sgl, "B":sgl}, "MB session out"=w323:refnum<class "MB_Master.lvclass">)  [unwired: 7 in]
              n135 = call "STD获取系列号.vi"("探头"=w322, "error in (no error)"=w324, "MB session in"=w323) -> ("error out"=w321:errorcluster, "SN"=w320:string)  [unwired: 6 in, 1 out]
              n136 = case shown="No Error" w321 {
                tunnel: w319 -> [w328 _]
                tunnel: w320 -> [w329 _]
                frame No Error {
                  n137 = Bundle("输出值"=w328, "SN"=w329) -> (w327:T5)  [unwired: 1 in]
                  n138 = global write "多参数全局变量.vi" "重新获取KB值命令"(FALSE ("重新获取KB值命令")) -> ()
                  n139 = global write "多参数全局变量.vi" "禹山KB值"(w327) -> ()
                }
                frame Error {
                }
              }
            }
          }
          n140 = global read "禹山过程全局变量.vi" "STDspcond"() -> (w315:cluster{"温度测量值":sgl, "测量值":sgl, "信号值":sgl})
          n141 = Unbundle By Name(w315) -> ("测量值"=w309:sgl, "信号值"=w305:sgl)
          n142 = Unbundle By Name(w312) -> ("K"=w310:sgl, "B"=w307:sgl)
        }
        frame "国弘" {
          n143 = global read "国弘过程全局变量.vi" "Cond"() -> (w345:T12)
          n144 = Unbundle By Name(w345) -> ("电导率测量值"=w344:sgl, "电导率信号值"=w343:sgl, "生产批次"=w336:u16, "电极序号"=w337:u16, "电导率电极零点"=w334:sgl, "电导率电极斜率"=w335:sgl, "温度补偿系数"=w333:sgl, "电极状态标志"=w331:u16)
          n145 = Number To Decimal String(number=w336) -> (decimal integer string=w342:string)  [unwired: 1 in]
          n146 = Number To Decimal String(number=w337) -> (decimal integer string=w340:string)  [unwired: 1 in]
          n147 = Concatenate Strings("MQ" ("字符串"), w342, "02" ("字符串"), w340) -> (w338:string)
        }
        frame "纳清" {
          n148 = global read "纳清过程全局变量.vi" "电导率测试值"() -> (w352:T13)
          n149 = Unbundle By Name(w352) -> ("电导率数据（uS/cm）"=w353:sgl, "电导率原始信号电阻"=w351:sgl, "序列号"=w350:string, "温度补偿系数"=w348:sgl)
        }
      }
    }
    frame 4 {
      n150 = Unbundle By Name(w362) -> ("叶绿素a探头选择"=w364:T1)
      n151 = case shown="\"禹山\", Default" w364 {
        tunnel: [w374 w399 w418 w424] -> w363
        tunnel: [w373 w390 w418 w422] -> w361
        tunnel: w360 -> [w371 w397 _ _]
        tunnel: [w372 w398 "" ("序列号") w421] -> w359
        tunnel: [w368 w394 _ _] -> w358
        tunnel: [w367 w393 _ _] -> w357
        tunnel: [_ _ TRUE TRUE] -> w356
        tunnel: ["%#.2f μg/L" ("数值文本.格式字符串") "%#.2f μg/L" ("数值文本.格式字符串") "%#.2f μg/L" ("数值文本.格式字符串") "%#.6f" ("数值文本.格式字符串")] -> w354
        frame "禹山", Default {
          n152 = global read "多参数全局变量.vi" "重新获取KB值命令"() -> (w365:bool)
          n153 = case shown="True" w365 {
            tunnel: [w376 w379] -> w372
            tunnel: w371 -> [_ w385]
            tunnel: [w377 w380] -> w370
            tunnel: T3."叶绿素a" ("探头") -> [_ w382]
            frame False {
              n154 = global read "多参数全局变量.vi" "禹山KB值"() -> (w378:T5)
              n155 = Unbundle By Name(w378) -> ("输出值"=w377:cluster{"K":sgl, "B":sgl}, "SN"=w376:string)
            }
            frame True {
              n156 = call "禹山获取用户校准参数.vi"("探头"=w382, "MB session in"=w385) -> ("error out"=w383:errorcluster, "输出值"=w380:cluster{"K":sgl, "B":sgl}, "MB session out"=w384:refnum<class "MB_Master.lvclass">)  [unwired: 7 in]
              n157 = call "禹山获取系列号.vi"("探头"=w382, "error in (no error)"=w383, "MB session in"=w384) -> ("error out"=w381:errorcluster, "SN"=w379:string)  [unwired: 6 in, 1 out]
              n158 = case shown="No Error" w381 {
                tunnel: w380 -> [w389 _]
                tunnel: w379 -> [w386 _]
                frame No Error {
                  n159 = Bundle("输出值"=w389, "SN"=w386) -> (w388:T5)  [unwired: 1 in]
                  n160 = global write "多参数全局变量.vi" "重新获取KB值命令"(FALSE ("重新获取KB值命令")) -> ()
                  n161 = global write "多参数全局变量.vi" "禹山KB值"(w388) -> ()
                }
                frame Error {
                }
              }
            }
          }
          n162 = global read "禹山过程全局变量.vi" "叶绿素a"() -> (w375:cluster{"温度测量值":sgl, "叶绿素测量值":sgl, "错误标志":u16})
          n163 = Unbundle By Name(w375) -> ("叶绿素测量值"=w374:sgl)
          n164 = Unbundle By Name(w370) -> ("K"=w368:sgl, "B"=w367:sgl)
          n165 = formula code="X = (Y-B)/K;"("Y"=w374, "K"=w368, "B"=w367) -> ("X"=w373:dbl)
        }
        frame "STD" {
          n166 = global read "多参数全局变量.vi" "重新获取KB值命令"() -> (w391:bool)
          n167 = case shown="True" w391 {
            tunnel: [w401 w404] -> w398
            tunnel: w397 -> [_ w410]
            tunnel: [w402 w405] -> w396
            tunnel: T3."叶绿素a" ("探头") -> [_ w407]
            frame False {
              n168 = global read "多参数全局变量.vi" "禹山KB值"() -> (w403:T5)
              n169 = Unbundle By Name(w403) -> ("输出值"=w402:cluster{"K":sgl, "B":sgl}, "SN"=w401:string)
            }
            frame True {
              n170 = call "STD获取用户校准参数.vi"("探头"=w407, "MB session in"=w410) -> ("error out"=w408:errorcluster, "输出值"=w405:cluster{"K":sgl, "B":sgl}, "MB session out"=w409:refnum<class "MB_Master.lvclass">)  [unwired: 7 in]
              n171 = call "STD获取系列号.vi"("探头"=w407, "error in (no error)"=w408, "MB session in"=w409) -> ("error out"=w406:errorcluster, "SN"=w404:string)  [unwired: 6 in, 1 out]
              n172 = case shown="No Error" w406 {
                tunnel: w405 -> [w414 _]
                tunnel: w404 -> [w411 _]
                frame No Error {
                  n173 = Bundle("输出值"=w414, "SN"=w411) -> (w413:T5)  [unwired: 1 in]
                  n174 = global write "多参数全局变量.vi" "重新获取KB值命令"(FALSE ("重新获取KB值命令")) -> ()
                  n175 = global write "多参数全局变量.vi" "禹山KB值"(w413) -> ()
                }
                frame Error {
                }
              }
            }
          }
          n176 = global read "禹山过程全局变量.vi" "STD叶绿素a"() -> (w400:cluster{"温度测量值":sgl, "叶绿素测量值":sgl, "信号值":sgl})
          n177 = Unbundle By Name(w400) -> ("叶绿素测量值"=w399:sgl, "信号值"=w390:sgl)
          n178 = Unbundle By Name(w396) -> ("K"=w394:sgl, "B"=w393:sgl)
        }
        frame "国弘" {
          w418 = sgl 0.0 ("温度数据")
        }
        frame "纳清" {
          n179 = global read "纳清过程全局变量.vi" "叶绿素a测试值"() -> (w423:T14)
          n180 = Unbundle By Name(w423) -> ("叶绿素a"=w424:sgl, "原始光强数值"=w422:u16, "序列号"=w421:string)
        }
      }
    }
    frame 5 {
      n181 = Unbundle By Name(w433) -> ("蓝绿藻探头选择"=w435:T1)
      n182 = case shown="\"STD\"" w435 {
        tunnel: [w439 w444 w469 w475] -> w434
        tunnel: [w439 w443 w469 w473] -> w432
        tunnel: ["" ("序列号") w440 "" ("序列号") w472] -> w431
        tunnel: [TRUE FALSE TRUE TRUE] -> w430
        tunnel: ["%#.2f cells/mL" ("数值文本.格式字符串") "%#.2f cells/mL" ("数值文本.格式字符串") "%#.2f cells/mL" ("数值文本.格式字符串") "%#.6f" ("数值文本.格式字符串")] -> w428
        tunnel: w427 -> [_ w445 _ _]
        tunnel: [_ w442 _ _] -> w426
        tunnel: [_ w441 _ _] -> w425
        frame "禹山", Default {
          w439 = sgl 0.0 ("温度数据")
        }
        frame "STD" {
          n183 = global read "多参数全局变量.vi" "重新获取KB值命令"() -> (w449:bool)
          n184 = case shown="True" w449 {
            tunnel: [w452 w455] -> w440
            tunnel: w445 -> [_ w461]
            tunnel: [w453 w456] -> w448
            tunnel: T4."藻密度" ("探头") -> [_ w458]
            frame False {
              n185 = global read "多参数全局变量.vi" "禹山KB值"() -> (w454:T5)
              n186 = Unbundle By Name(w454) -> ("输出值"=w453:cluster{"K":sgl, "B":sgl}, "SN"=w452:string)
            }
            frame True {
              n187 = call "STD获取用户校准参数.vi"("探头"=w458, "MB session in"=w461) -> ("error out"=w459:errorcluster, "输出值"=w456:cluster{"K":sgl, "B":sgl}, "MB session out"=w460:refnum<class "MB_Master.lvclass">)  [unwired: 7 in]
              n188 = call "STD获取系列号.vi"("探头"=w458, "error in (no error)"=w459, "MB session in"=w460) -> ("error out"=w457:errorcluster, "SN"=w455:string)  [unwired: 6 in, 1 out]
              n189 = case shown="No Error" w457 {
                tunnel: w456 -> [w465 _]
                tunnel: w455 -> [w462 _]
                frame No Error {
                  n190 = Bundle("输出值"=w465, "SN"=w462) -> (w464:T5)  [unwired: 1 in]
                  n191 = global write "多参数全局变量.vi" "重新获取KB值命令"(FALSE ("重新获取KB值命令")) -> ()
                  n192 = global write "多参数全局变量.vi" "禹山KB值"(w464) -> ()
                }
                frame Error {
                }
              }
            }
          }
          n193 = global read "禹山过程全局变量.vi" "STD藻密度"() -> (w447:cluster{"温度测量值":sgl, "测量值":sgl, "信号值":sgl})
          n194 = Unbundle By Name(w447) -> ("测量值"=w444:sgl, "信号值"=w443:sgl)
          n195 = Unbundle By Name(w448) -> ("K"=w442:sgl, "B"=w441:sgl)
        }
        frame "国弘" {
          w469 = sgl 0.0 ("温度数据")
        }
        frame "纳清" {
          n196 = global read "纳清过程全局变量.vi" "蓝绿藻测试值"() -> (w474:T15)
          n197 = Unbundle By Name(w474) -> ("蓝绿藻"=w475:sgl, "原始光强数值"=w473:u16, "序列号"=w472:string)
        }
      }
    }
    frame 6 {
      n198 = Unbundle By Name(w484) -> ("orp探头选择"=w486:T1)
      n199 = case shown="\"禹山\", Default" w486 {
        tunnel: [w489 w500 w504] -> w485
        tunnel: [w489 w499 w504] -> w483
        tunnel: ["" w492 ""] -> w482
        tunnel: [TRUE TRUE TRUE] -> w481
        tunnel: [_ w490 _] -> w477
        frame "禹山", Default {
          w489 = sgl 0.0 ("温度数据")
        }
        frame "国弘" {
          n200 = global read "国弘过程全局变量.vi" "ORP"() -> (w501:T16)
          n201 = Unbundle By Name(w501) -> ("测量值"=w500:sgl, "信号值"=w499:sgl, "生产批次"=w493:u16, "传感器序号"=w494:u16, "电极状态标志"=w490:u16)
          n202 = Number To Decimal String(number=w493) -> (decimal integer string=w498:string)  [unwired: 1 in]
          n203 = Number To Decimal String(number=w494) -> (decimal integer string=w496:string)  [unwired: 1 in]
          n204 = Concatenate Strings("MQ" ("字符串"), w498, "05" ("字符串"), w496) -> (w492:string)
        }
        frame "纳清" {
          w504 = sgl 0.0 ("温度测量值")
        }
      }
    }
    frame 7 {
      n205 = global read "国弘过程全局变量.vi" "COD"() -> (w511:T17)
      n206 = Unbundle By Name(w511) -> ("电极状态标志"=w513:u16, "COD测量值"=w519:sgl, "COD信号值"=w518:sgl, "生产批次"=w506:u16, "电极序号"=w505:u16, "COD零点系数"=w515:sgl, "COD斜率系数"=w516:sgl)
      n207 = Number To Decimal String(number=w506) -> (decimal integer string=w510:string)  [unwired: 1 in]
      n208 = Number To Decimal String(number=w505) -> (decimal integer string=w508:string)  [unwired: 1 in]
      n209 = Concatenate Strings("MQ" ("字符串"), w510, "08" ("字符串"), w508) -> (w517:string)
    }
    frame 8 {
      n210 = global read "多参数全局变量.vi" "重新获取KB值命令"() -> (w520:bool)
      n211 = case shown="False" w520 {
        tunnel: [w534 w536] -> w529
        tunnel: w528 -> [_ w542]
        tunnel: [w533 w537] -> w527
        tunnel: T3."DO2" ("探头") -> [_ w539]
        frame False {
          n212 = global read "多参数全局变量.vi" "禹山KB值"() -> (w535:T5)
          n213 = Unbundle By Name(w535) -> ("输出值"=w533:cluster{"K":sgl, "B":sgl}, "SN"=w534:string)
        }
        frame True {
          n214 = call "禹山获取用户校准参数.vi"("探头"=w539, "MB session in"=w542) -> ("error out"=w541:errorcluster, "输出值"=w537:cluster{"K":sgl, "B":sgl}, "MB session out"=w540:refnum<class "MB_Master.lvclass">)  [unwired: 7 in]
          n215 = call "禹山获取系列号.vi"("探头"=w539, "error in (no error)"=w541, "MB session in"=w540) -> ("error out"=w538:errorcluster, "SN"=w536:string)  [unwired: 6 in, 1 out]
          n216 = case shown="No Error" w538 {
            tunnel: w537 -> [w545 _]
            tunnel: w536 -> [w546 _]
            frame No Error {
              n217 = Bundle("输出值"=w545, "SN"=w546) -> (w544:T5)  [unwired: 1 in]
              n218 = global write "多参数全局变量.vi" "重新获取KB值命令"(FALSE ("重新获取KB值命令")) -> ()
              n219 = global write "多参数全局变量.vi" "禹山KB值"(w544) -> ()
            }
            frame Error {
            }
          }
        }
      }
      n220 = global read "禹山过程全局变量.vi" "DO 2"() -> (w532:cluster{"温度测量值":sgl, "DO%":sgl, "DOmg/L":sgl})
      n221 = Unbundle By Name(w532) -> ("DO%"=w530:sgl)
      n222 = Unbundle By Name(w527) -> ("K"=w524:sgl, "B"=w523:sgl)
      n223 = formula code="Y = Y / 100;\nX = (Y-B)/K;\nX = 100 * X;"("Y"=w530, "K"=w524, "B"=w523) -> ("X"=w531:dbl)
    }
    frame 9 {
      n224 = global read "国弘过程全局变量.vi" "氯化物"() -> (w553:T18)
      n225 = Unbundle By Name(w553) -> ("电极状态标志"=w555:u16, "测量值"=w561:sgl, "信号值"=w560:sgl, "生产批次"=w548:u16, "电极序号"=w547:u16, "电极零点"=w557:sgl, "电极斜率"=w558:sgl)
      n226 = Number To Decimal String(number=w548) -> (decimal integer string=w552:string)  [unwired: 1 in]
      n227 = Number To Decimal String(number=w547) -> (decimal integer string=w550:string)  [unwired: 1 in]
      n228 = Concatenate Strings("MQ" ("字符串"), w552, "01" ("字符串"), w550) -> (w559:string)
    }
    frame 10 {
      n229 = global read "纳清过程全局变量.vi" "氨氮测试值"() -> (w562:T19)
      n230 = Unbundle By Name(w562) -> ("参数2数据"=w568:sgl, "参数2原始信号"=w567:sgl, "序列号"=w566:string)
    }
    frame 11 {
      n231 = global read "国弘过程全局变量.vi" "水中油"() -> (w575:T20)
      n232 = Unbundle By Name(w575) -> ("电极状态标志"=w577:u16, "测量值"=w583:sgl, "信号值"=w582:sgl, "生产批次"=w570:u16, "电极序号"=w569:u16, "水中油零点系数"=w579:sgl, "水中油斜率系数"=w580:sgl)
      n233 = Number To Decimal String(number=w570) -> (decimal integer string=w574:string)  [unwired: 1 in]
      n234 = Number To Decimal String(number=w569) -> (decimal integer string=w572:string)  [unwired: 1 in]
      n235 = Concatenate Strings("MQ" ("字符串"), w574, "17" ("字符串"), w572) -> (w581:string)
    }
  }
  "检测值" <- w17
  "信号值" <- w14
  "序列号" <- w12
  "检测值.格式字符串" <- w6
  "电极状态标志" <- w2
  "信号值.格式字符串" <- w1
  n236 = Not(x=w11) -> (.not. x?=w10:bool)
  n237 = Bundle(w5, "温度补偿系数"=w4) -> (→"温度补偿系数":cluster{bool, "温度补偿系数":sgl})  [unwired: 1 in]
  n238 = Bundle(w10, "水中油斜率系数"=w9, "水中油零点系数"=w8) -> (→"线性系数":cluster{bool, "水中油斜率系数":sgl, "水中油零点系数":sgl})  [unwired: 1 in]
